vi "AlazarWaitNextAsyncBufferCompleteI16.vi"(4 "bytesToCopy":u32, 5 "timeout_ms":u32, 6 "Buffer":u16[](array[numeric]), 7 "Handle":u32) -> (1 "Return Code":u32, 2 "Buffer":u16[](array[numeric]), 3 "Handle":u32)   [LabVIEW 2024]
doc: "This function returns when the board has received sufficient trigger events to fill the buffer, or the timeout interval has elapsed. To use this function, AlazarBeforeAsyncRead must be called with the ADMA_ALLOC_BUFFERS flag."
uses:
  ATSApi.dll
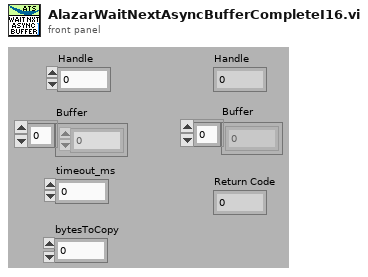
[diagram p1: front panel]
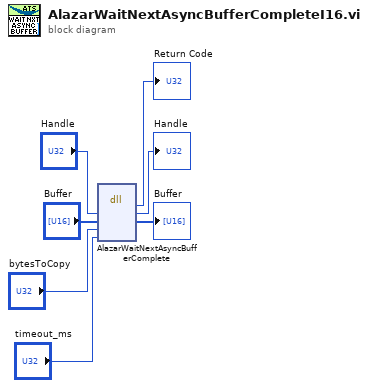
[diagram p0: block diagram]
diagram:
  n1 = dll-call lib="ATSApi.dll" fn="AlazarWaitNextAsyncBufferComplete"("handle"="Handle", "buffer"="Buffer", "bytesToCopy"="bytesToCopy", "timeout_ms"="timeout_ms") -> ("return type"=→"Return Code":u32, "handle"=→"Handle":u32, "buffer"=→"Buffer":u16[])  [unwired: 5 in, 2 out]
